vi "Change_Parameter.vi"(0 "Spinal Column In":T1={"Red MOT 88 Inputs"={"Active Device"="", "Active Channels"=[], "Waveform Parameters"=[], "Active Phases"=[], "Phase Times"=[], "Trigger Channel"=""}, "6704 Static Voltage Settings"={"Device Name"="", "Values"=[], "Nickname"=[], "Conversion"=[]}, "Instructions"=[], "Red MOT 87 Inputs"={"Active Device"="", "Active Channels"=[], "Waveform Parameters"=[], "Active Phases"=[], "Phase Times"=[], "Trigger Channel"=""}, "ODT Params"={"Waveform Parameters"=[], "Active Phases"=[], "Active Channels"=[], "Phase Times (s)"=[], "Active Device"="", "Trigger Channel"="", "Evaporation Phase"=0.0, "Evaporation Channel"=0.0}, "SR400 Settings"={"Channel A"={"Input"=0, "A Discriminator Level (V)"=0.0, "A Discriminator Slope"=enum."Rising", "A Gate Mode"=enum."CW", "A Gate Delay (s)"=0.0, "A Gate Width (s)"=0.0, "Scan Increment (s)"=0.0}, "Channel B"={"Input"=0, "B Discriminator Level (V)"=0.0, "B Discriminator Slope"=enum."Rising", "B Gate Mode"=enum."CW", "B Gate Delay (s)"=0.0, "B Gate Width (s)"=0.0, "Scan Increment (s)"=0.0}, "Channel T"={"Input"=0, "Trigger Level (V)"=0.0, "Trigger Slope"=enum."Rising", "T Discriminator Slope"=enum."Rising", "T Discriminator Level (V)"=0.0, "Trigger Preset"=0.0}, "N Periods"=0.0, "At N"=enum."Stop", "Counting Mode"=enum."A,B for T Preset", "GPIB Address"="", "Dwell Time (s)"=0.0, "Port 1 Mode"=0, "Port 1 Voltage"=0.0, "Port 1 Scan Increment"=0.0, "Port 2 Voltage"=0.0, "Port 2 Scan Increment"=0.0, "Port 2 Mode"=0, "Counter Toggle"=FALSE, "Pusleblater Settings"={"Loop Start Channel"=0.0, "Loop End Channel"=0.0, "Loop On"=FALSE}}, "Synth Controls"={"Channel Settings"=[], "Active Channels"=[], "COM Port"=""}, "Acquisition Parameters"={"Acquisition Mode"=enum."Reserved (0)", "Trigger Mode"=enum."Internal", "Frame \nTransfer"=FALSE, "Exposure Time (s)"=0.0, "Accumulation Cycle Time (s)"=0.0, "# Accumulations"=0, "# Kinetics"=0, "Kinetic Cycle Time (s)"=0.0, "Horizontal Bin Size"=0, "Vertical Bin Size"=0}, "Scan Parameters"={"Initial Values"=[], "Final Values"=[], "Step Sizes"=[], "Parameters to Change"=[], "Channels to Change"=[], "Number of Parameters to Scan"=0, "Parameter Nickname (no spaces)"=[], "Scan Base Name"="", "Raw_Data Folder"=path "", "ROI Parameters"={"Background Radius"=0.0, "Atom Radius"=0.0, "X Center"=0.0, "Y Center"=0.0}, "Drop Time (ms)"=0.0, "ODT VCA 1 Channel"=0.0, "ODT VCA 2 Channel"=0.0, "Phases To Change"=[], "Scan Pulseblaster Channel With Parameter"={"Change PB Time Toggle"=FALSE, "PB Channel"=0.0, "Parameter Number"=0.0}, "Preserve Waveform\nContinuity"=FALSE, "Generated Array Type"=enum."Custom Array From File", "Principle Quantum #"=0, "Angular Momentum"=enum."s", "Ramp Delay Channel"=0, "ODT Hold Channel"=0, "MCS ROI Min"=0, "MCS ROI Max"=0, "Master Batch Fourth Column"=0.0}, "MCS Parameters"={"Scan Length (Bins)"=0.0, "Dwell Time (s)"=0.0, "Gate Channel Settings"={"Threshold (V)"=0.0, "Edge"=enum."Falling", "Input Impedence"=enum."1k Ohm"}, "Trig Channel Settings"={"Threshold (V)"=0.0, "Edge"=enum."Falling", "Input Impedence"=enum."1k Ohm"}, "Input 1 Settings"={"Threshold (V)"=0.0, "Edge"=enum."Falling", "Input Impedence"=enum."1k Ohm"}, "Input 2 Settings"={"Threshold (V)"=0.0, "Edge"=enum."Falling", "Input Impedence"=enum."1k Ohm"}, "Number of Sweeps"=0, "Number of Sequential Cycles"=0.0, "Number of Sequences"=0.0, "Sweep Preset"=FALSE, "Sequential Mode"=FALSE, "DAC 1 Ramp Settings"={"Ramp Mode"=enum."Fixed", "Ramp Start Value (V)"=0.0, "Ramp Length (Steps)"=0, "Step Width (bins)"=0, "Step Size (V)"=0.0}, "DAC 2 Output (V)"=0.0, "SYNC Output"=enum."40 MHz Clock", "ROI Min"=0, "ROI Max"=0, "Dual MCS Mode"=FALSE, "DAC 2 Toggle"=FALSE, "MCS on/off"=FALSE, "ROI Max 2"=1, "ROI Min 2"=0}, "PicoScope"={"Channel A Settings"={"Enabled"=FALSE, "Coupling"=0, "Range"=0, "Analogue Offset"=0.0}, "Channel B Settings"={"Enabled"=FALSE, "Coupling"=0, "Range"=0, "Analogue Offset"=0.0}, "Trigger Options"={"Trigger Enabled"=FALSE, "Trigger Source"=enum."Channel A", "Trigger Threshold (-5 to 5 V)"=0.0, "Trigger Slope"=0, "Trigger Delay (ms)"=0.0, "Auto Trigger Time (ms)"=0}, "Pico Scope Inititalization Settings"={"USB Power"=FALSE, "Use Serial Number"=FALSE, "Resolution"=0, "Serial Number"="", "Handle"=0}, "Use PicoScope?"=FALSE, "Acquisition Settings"={"Pre Trigger Time (s)"=0.0, "Post Trigger Time (s)"=0.0, "Resolution (s)"=0.0, "Four Channel Device"=FALSE, "Number of Captures"=0.0}}, "Random Interleave Controls"={"Subroutine A"=[], "Subroutine B"=[], "Interleave On"=FALSE, "Number of loops"=0, "Insert after instruction"=0, "Random"=FALSE}} {"Red MOT 88 Inputs"."Phase Times" format="%.0p"; "Red MOT 87 Inputs"."Phase Times" format="%.0p"; "ODT Params"."Evaporation Channel" min=0.0 max=1.0 step=1.0; "ODT Params"."Evaporation Phase" min=0.0 max=4.0 step=1.0; "ODT Params"."Phase Times (s)" format="%#_6p"; "SR400 Settings"."Port 2 Mode" items=["Scan"=1, "Fixed"=0]; "SR400 Settings"."Port 2 Scan Increment" min=-0.5 max=0.5; "SR400 Settings"."Port 2 Voltage" min=-10.0 max=10.0; "SR400 Settings"."Port 1 Scan Increment" min=-0.5 max=-0.5; "SR400 Settings"."Port 1 Voltage" min=-10.0 max=10.0; "SR400 Settings"."Port 1 Mode" items=["Scan"=1, "Fixed"=0]; "SR400 Settings"."Dwell Time (s)" min=0.002 max=60.0 format="%#_6p"; "SR400 Settings"."N Periods" min=1.0 max=2000.0 step=1.0; "SR400 Settings"."Channel T"."Trigger Preset" min=1.0 max=900000000000.0 format="%#_1e"; "SR400 Settings"."Channel T"."T Discriminator Level (V)" min=-0.3 max=0.3 format="%#_6p"; "SR400 Settings"."Channel T"."Trigger Level (V)" min=-2.0 max=2.0 format="%#_6p"; "SR400 Settings"."Channel T"."Input" items=["10 MHz", "Input 2", "Trig"]; "SR400 Settings"."Channel B"."Scan Increment (s)" min=0.0 max=0.09992 format="%#_6p"; "SR400 Settings"."Channel B"."B Gate Width (s)" min=5e-09 max=0.9992 format="%#_6p"; "SR400 Settings"."Channel B"."B Gate Delay (s)" min=0.0 max=0.9992 format="%#_6p"; "SR400 Settings"."Channel B"."B Discriminator Level (V)" min=-0.3 max=0.3 format="%#_6p"; "SR400 Settings"."Channel B"."Input" items=["Input 2"=2, "Input 1"=1]; "SR400 Settings"."Channel A"."Scan Increment (s)" min=0.0 max=0.09992 format="%#_6p"; "SR400 Settings"."Channel A"."A Gate Width (s)" min=5e-09 max=0.9992 format="%#_6p"; "SR400 Settings"."Channel A"."A Gate Delay (s)" min=0.0 max=0.9992 format="%#_6p"; "SR400 Settings"."Channel A"."A Discriminator Level (V)" min=-0.3 max=0.3 format="%#_6p"; "SR400 Settings"."Channel A"."Input" items=["Input 1", "10 MHz"]; "Acquisition Parameters"."Vertical Bin Size" items=["6"=6, "3"=3, "2"=2, "1"=1]; "Acquisition Parameters"."Horizontal Bin Size" items=["4"=4, "2"=2, "1"=1]; "Acquisition Parameters"."Kinetic Cycle Time (s)" format="%.2f"; "Acquisition Parameters"."# Kinetics" min=1; "Acquisition Parameters"."# Accumulations" min=1; "Acquisition Parameters"."Accumulation Cycle Time (s)" format="%.2f"; "Acquisition Parameters"."Exposure Time (s)" format="%.2f"; "Scan Parameters"."Drop Time (ms)" min=1.0; "Scan Parameters"."Number of Parameters to Scan" min=1; "MCS Parameters"."ROI Max 2" min=1; "MCS Parameters"."ROI Min 2" min=0; "MCS Parameters"."ROI Max" min=1; "MCS Parameters"."ROI Min" min=0; "MCS Parameters"."DAC 2 Output (V)" min=-10.0 max=10.0 step=0.00488; "MCS Parameters"."DAC 1 Ramp Settings"."Step Size (V)" min=0.0 max=10.0 step=0.00244 format="%#_4g"; "MCS Parameters"."DAC 1 Ramp Settings"."Step Width (bins)" min=1; "MCS Parameters"."DAC 1 Ramp Settings"."Ramp Length (Steps)" min=1; "MCS Parameters"."DAC 1 Ramp Settings"."Ramp Start Value (V)" min=0.0 max=10.0 step=0.00244; "MCS Parameters"."Number of Sweeps" min=0 format="%.0p"; "MCS Parameters"."Input 2 Settings"."Threshold (V)" min=-2.5 max=2.5 step=0.001; "MCS Parameters"."Input 1 Settings"."Threshold (V)" min=-2.5 max=2.5 step=0.001; "MCS Parameters"."Trig Channel Settings"."Threshold (V)" min=-2.5 max=2.5 step=0.001; "MCS Parameters"."Gate Channel Settings"."Threshold (V)" min=-2.5 max=2.5 step=0.001; "MCS Parameters"."Dwell Time (s)" min=1e-07 step=2.5e-08 format="%#_6p"; "MCS Parameters"."Scan Length (Bins)" min=64.0 max=524288.0 format="%#_7f"; "PicoScope"."Acquisition Settings"."Resolution (s)" min=8e-09 max=34.36 step=8e-09 format="%#_6p"; "PicoScope"."Acquisition Settings"."Post Trigger Time (s)" min=0.0 format="%#_6p"; "PicoScope"."Acquisition Settings"."Pre Trigger Time (s)" min=0.0 format="%#_6p"; "PicoScope"."Pico Scope Inititalization Settings"."Resolution" items=["8-bit", "12-bit", "14-bit", "15-bit (max. 2 ch.)", "16-bit (max. 1 ch.)"]; "PicoScope"."Trigger Options"."Trigger Slope" items=["Rising"=2, "Falling"=3]; "PicoScope"."Channel B Settings"."Range" items=["10 mV", "20 mV", "50 mV", "100 mV", "200 mV", "500 mV", "1 V", "2 V", "5 V", "10 V", "20 V", "50 V ", "100 V"]; "PicoScope"."Channel B Settings"."Coupling" items=["AC", "DC"]; "PicoScope"."Channel A Settings"."Range" items=["10 mV", "20 mV", "50 mV", "100 mV", "200 mV", "500 mV", "1 V", "2 V", "5 V", "10 V", "20 V", "50 V ", "100 V"]; "PicoScope"."Channel A Settings"."Coupling" items=["AC", "DC"]; "Random Interleave Controls"."Insert after instruction" min=0; "Random Interleave Controls"."Subroutine B"."Time (s)" min=5e-08 format="%.3p"; "Random Interleave Controls"."Subroutine B"."Op Code" items=["Continue", "Stop", "Loop", "End Loop", "JSR", "RTS", "Branch", "Long Delay", "Wait"]; "Random Interleave Controls"."Subroutine B"."Instruct Data" format="%.0p"; "Random Interleave Controls"."Subroutine A"."Time (s)" min=5e-08 format="%.3p"; "Random Interleave Controls"."Subroutine A"."Op Code" items=["Continue", "Stop", "Loop", "End Loop", "JSR", "RTS", "Branch", "Long Delay", "Wait"]; "Random Interleave Controls"."Subroutine A"."Instruct Data" format="%.0p"}, 5 "What To Change":T25=enum."Synth Frequency", 7 "Channel To Change":dbl, 9 "Phase To Change":dbl, 11 "Value":dbl, 12 "Scan Pulseblaster Channel With Parameter":T27, 13 "Current Parameter":i32, 14 "Waveform Continuity":bool) -> (6 "Spinal Column Out":T1={"Red MOT 88 Inputs"={"Active Device"="", "Active Channels"=[], "Waveform Parameters"=[], "Active Phases"=[], "Phase Times"=[], "Trigger Channel"=""}, "6704 Static Voltage Settings"={"Device Name"="", "Values"=[], "Nickname"=[], "Conversion"=[]}, "Instructions"=[], "Red MOT 87 Inputs"={"Active Device"="", "Active Channels"=[], "Waveform Parameters"=[], "Active Phases"=[], "Phase Times"=[], "Trigger Channel"=""}, "ODT Params"={"Waveform Parameters"=[], "Active Phases"=[], "Active Channels"=[], "Phase Times (s)"=[], "Active Device"="", "Trigger Channel"="", "Evaporation Phase"=0.0, "Evaporation Channel"=0.0}, "SR400 Settings"={"Channel A"={"Input"=0, "A Discriminator Level (V)"=0.0, "A Discriminator Slope"=enum."Rising", "A Gate Mode"=enum."CW", "A Gate Delay (s)"=0.0, "A Gate Width (s)"=0.0, "Scan Increment (s)"=0.0}, "Channel B"={"Input"=0, "B Discriminator Level (V)"=0.0, "B Discriminator Slope"=enum."Rising", "B Gate Mode"=enum."CW", "B Gate Delay (s)"=0.0, "B Gate Width (s)"=0.0, "Scan Increment (s)"=0.0}, "Channel T"={"Input"=0, "Trigger Level (V)"=0.0, "Trigger Slope"=enum."Rising", "T Discriminator Slope"=enum."Rising", "T Discriminator Level (V)"=0.0, "Trigger Preset"=0.0}, "N Periods"=0.0, "At N"=enum."Stop", "Counting Mode"=enum."A,B for T Preset", "GPIB Address"="", "Dwell Time (s)"=0.0, "Port 1 Mode"=0, "Port 1 Voltage"=0.0, "Port 1 Scan Increment"=0.0, "Port 2 Voltage"=0.0, "Port 2 Scan Increment"=0.0, "Port 2 Mode"=0, "Counter Toggle"=FALSE, "Pusleblater Settings"={"Loop Start Channel"=0.0, "Loop End Channel"=0.0, "Loop On"=FALSE}}, "Synth Controls"={"Channel Settings"=[], "Active Channels"=[], "COM Port"=""}, "Acquisition Parameters"={"Acquisition Mode"=enum."Reserved (0)", "Trigger Mode"=enum."Internal", "Frame \nTransfer"=FALSE, "Exposure Time (s)"=0.0, "Accumulation Cycle Time (s)"=0.0, "# Accumulations"=0, "# Kinetics"=0, "Kinetic Cycle Time (s)"=0.0, "Horizontal Bin Size"=0, "Vertical Bin Size"=0}, "Scan Parameters"={"Initial Values"=[], "Final Values"=[], "Step Sizes"=[], "Parameters to Change"=[], "Channels to Change"=[], "Number of Parameters to Scan"=0, "Parameter Nickname (no spaces)"=[], "Scan Base Name"="", "Raw_Data Folder"=path "", "ROI Parameters"={"Background Radius"=0.0, "Atom Radius"=0.0, "X Center"=0.0, "Y Center"=0.0}, "Drop Time (ms)"=0.0, "ODT VCA 1 Channel"=0.0, "ODT VCA 2 Channel"=0.0, "Phases To Change"=[], "Scan Pulseblaster Channel With Parameter"={"Change PB Time Toggle"=FALSE, "PB Channel"=0.0, "Parameter Number"=0.0}, "Preserve Waveform\nContinuity"=FALSE, "Generated Array Type"=enum."Custom Array From File", "Principle Quantum #"=0, "Angular Momentum"=enum."s", "Ramp Delay Channel"=0, "ODT Hold Channel"=0, "MCS ROI Min"=0, "MCS ROI Max"=0, "Master Batch Fourth Column"=0.0}, "MCS Parameters"={"Scan Length (Bins)"=0.0, "Dwell Time (s)"=0.0, "Gate Channel Settings"={"Threshold (V)"=0.0, "Edge"=enum."Falling", "Input Impedence"=enum."1k Ohm"}, "Trig Channel Settings"={"Threshold (V)"=0.0, "Edge"=enum."Falling", "Input Impedence"=enum."1k Ohm"}, "Input 1 Settings"={"Threshold (V)"=0.0, "Edge"=enum."Falling", "Input Impedence"=enum."1k Ohm"}, "Input 2 Settings"={"Threshold (V)"=0.0, "Edge"=enum."Falling", "Input Impedence"=enum."1k Ohm"}, "Number of Sweeps"=0, "Number of Sequential Cycles"=0.0, "Number of Sequences"=0.0, "Sweep Preset"=FALSE, "Sequential Mode"=FALSE, "DAC 1 Ramp Settings"={"Ramp Mode"=enum."Fixed", "Ramp Start Value (V)"=0.0, "Ramp Length (Steps)"=0, "Step Width (bins)"=0, "Step Size (V)"=0.0}, "DAC 2 Output (V)"=0.0, "SYNC Output"=enum."40 MHz Clock", "ROI Min"=0, "ROI Max"=0, "Dual MCS Mode"=FALSE, "DAC 2 Toggle"=FALSE, "MCS on/off"=FALSE, "ROI Max 2"=1, "ROI Min 2"=0}, "PicoScope"={"Channel A Settings"={"Enabled"=FALSE, "Coupling"=0, "Range"=0, "Analogue Offset"=0.0}, "Channel B Settings"={"Enabled"=FALSE, "Coupling"=0, "Range"=0, "Analogue Offset"=0.0}, "Trigger Options"={"Trigger Enabled"=FALSE, "Trigger Source"=enum."Channel A", "Trigger Threshold (-5 to 5 V)"=0.0, "Trigger Slope"=0, "Trigger Delay (ms)"=0.0, "Auto Trigger Time (ms)"=0}, "Pico Scope Inititalization Settings"={"USB Power"=FALSE, "Use Serial Number"=FALSE, "Resolution"=0, "Serial Number"="", "Handle"=0}, "Use PicoScope?"=FALSE, "Acquisition Settings"={"Pre Trigger Time (s)"=0.0, "Post Trigger Time (s)"=0.0, "Resolution (s)"=0.0, "Four Channel Device"=FALSE, "Number of Captures"=0.0}}, "Random Interleave Controls"={"Subroutine A"=[], "Subroutine B"=[], "Interleave On"=FALSE, "Number of loops"=0, "Insert after instruction"=0, "Random"=FALSE}} {"Red MOT 88 Inputs"."Phase Times" format="%.0p"; "Red MOT 87 Inputs"."Phase Times" format="%.0p"; "ODT Params"."Evaporation Channel" min=0.0 max=1.0 step=1.0; "ODT Params"."Evaporation Phase" min=0.0 max=4.0 step=1.0; "ODT Params"."Phase Times (s)" format="%#_6p"; "SR400 Settings"."Port 2 Mode" items=["Scan"=1, "Fixed"=0]; "SR400 Settings"."Port 2 Scan Increment" min=-0.5 max=0.5; "SR400 Settings"."Port 2 Voltage" min=-10.0 max=10.0; "SR400 Settings"."Port 1 Scan Increment" min=-0.5 max=-0.5; "SR400 Settings"."Port 1 Voltage" min=-10.0 max=10.0; "SR400 Settings"."Port 1 Mode" items=["Scan"=1, "Fixed"=0]; "SR400 Settings"."Dwell Time (s)" min=0.002 max=60.0 format="%#_6p"; "SR400 Settings"."N Periods" min=1.0 max=2000.0 step=1.0; "SR400 Settings"."Channel T"."Trigger Preset" min=1.0 max=900000000000.0 format="%#_1e"; "SR400 Settings"."Channel T"."T Discriminator Level (V)" min=-0.3 max=0.3 format="%#_6p"; "SR400 Settings"."Channel T"."Trigger Level (V)" min=-2.0 max=2.0 format="%#_6p"; "SR400 Settings"."Channel T"."Input" items=["10 MHz", "Input 2", "Trig"]; "SR400 Settings"."Channel B"."Scan Increment (s)" min=0.0 max=0.09992 format="%#_6p"; "SR400 Settings"."Channel B"."B Gate Width (s)" min=5e-09 max=0.9992 format="%#_6p"; "SR400 Settings"."Channel B"."B Gate Delay (s)" min=0.0 max=0.9992 format="%#_6p"; "SR400 Settings"."Channel B"."B Discriminator Level (V)" min=-0.3 max=0.3 format="%#_6p"; "SR400 Settings"."Channel B"."Input" items=["Input 2"=2, "Input 1"=1]; "SR400 Settings"."Channel A"."Scan Increment (s)" min=0.0 max=0.09992 format="%#_6p"; "SR400 Settings"."Channel A"."A Gate Width (s)" min=5e-09 max=0.9992 format="%#_6p"; "SR400 Settings"."Channel A"."A Gate Delay (s)" min=0.0 max=0.9992 format="%#_6p"; "SR400 Settings"."Channel A"."A Discriminator Level (V)" min=-0.3 max=0.3 format="%#_6p"; "SR400 Settings"."Channel A"."Input" items=["Input 1", "10 MHz"]; "Acquisition Parameters"."Vertical Bin Size" items=["6"=6, "3"=3, "2"=2, "1"=1]; "Acquisition Parameters"."Horizontal Bin Size" items=["4"=4, "2"=2, "1"=1]; "Acquisition Parameters"."Kinetic Cycle Time (s)" format="%.2f"; "Acquisition Parameters"."# Kinetics" min=1; "Acquisition Parameters"."# Accumulations" min=1; "Acquisition Parameters"."Accumulation Cycle Time (s)" format="%.2f"; "Acquisition Parameters"."Exposure Time (s)" format="%.2f"; "Scan Parameters"."Drop Time (ms)" min=1.0; "Scan Parameters"."Number of Parameters to Scan" min=1; "MCS Parameters"."ROI Max 2" min=1; "MCS Parameters"."ROI Min 2" min=0; "MCS Parameters"."ROI Max" min=1; "MCS Parameters"."ROI Min" min=0; "MCS Parameters"."DAC 2 Output (V)" min=-10.0 max=10.0 step=0.00488; "MCS Parameters"."DAC 1 Ramp Settings"."Step Size (V)" min=0.0 max=10.0 step=0.00244 format="%#_4g"; "MCS Parameters"."DAC 1 Ramp Settings"."Step Width (bins)" min=1; "MCS Parameters"."DAC 1 Ramp Settings"."Ramp Length (Steps)" min=1; "MCS Parameters"."DAC 1 Ramp Settings"."Ramp Start Value (V)" min=0.0 max=10.0 step=0.00244; "MCS Parameters"."Number of Sweeps" min=0 format="%.0p"; "MCS Parameters"."Input 2 Settings"."Threshold (V)" min=-2.5 max=2.5 step=0.001; "MCS Parameters"."Input 1 Settings"."Threshold (V)" min=-2.5 max=2.5 step=0.001; "MCS Parameters"."Trig Channel Settings"."Threshold (V)" min=-2.5 max=2.5 step=0.001; "MCS Parameters"."Gate Channel Settings"."Threshold (V)" min=-2.5 max=2.5 step=0.001; "MCS Parameters"."Dwell Time (s)" min=1e-07 step=2.5e-08 format="%#_6p"; "MCS Parameters"."Scan Length (Bins)" min=64.0 max=524288.0 format="%#_7f"; "PicoScope"."Acquisition Settings"."Resolution (s)" min=8e-09 max=34.36 step=8e-09 format="%#_6p"; "PicoScope"."Acquisition Settings"."Post Trigger Time (s)" min=0.0 format="%#_6p"; "PicoScope"."Acquisition Settings"."Pre Trigger Time (s)" min=0.0 format="%#_6p"; "PicoScope"."Pico Scope Inititalization Settings"."Resolution" items=["8-bit", "12-bit", "14-bit", "15-bit (max. 2 ch.)", "16-bit (max. 1 ch.)"]; "PicoScope"."Trigger Options"."Trigger Slope" items=["Rising"=2, "Falling"=3]; "PicoScope"."Channel B Settings"."Range" items=["10 mV", "20 mV", "50 mV", "100 mV", "200 mV", "500 mV", "1 V", "2 V", "5 V", "10 V", "20 V", "50 V ", "100 V"]; "PicoScope"."Channel B Settings"."Coupling" items=["AC", "DC"]; "PicoScope"."Channel A Settings"."Range" items=["10 mV", "20 mV", "50 mV", "100 mV", "200 mV", "500 mV", "1 V", "2 V", "5 V", "10 V", "20 V", "50 V ", "100 V"]; "PicoScope"."Channel A Settings"."Coupling" items=["AC", "DC"]; "Random Interleave Controls"."Insert after instruction" min=0; "Random Interleave Controls"."Subroutine B"."Time (s)" min=5e-08 format="%.3p"; "Random Interleave Controls"."Subroutine B"."Op Code" items=["Continue", "Stop", "Loop", "End Loop", "JSR", "RTS", "Branch", "Long Delay", "Wait"]; "Random Interleave Controls"."Subroutine B"."Instruct Data" format="%.0p"; "Random Interleave Controls"."Subroutine A"."Time (s)" min=5e-08 format="%.3p"; "Random Interleave Controls"."Subroutine A"."Op Code" items=["Continue", "Stop", "Loop", "End Loop", "JSR", "RTS", "Branch", "Long Delay", "Wait"]; "Random Interleave Controls"."Subroutine A"."Instruct Data" format="%.0p"}, 10 "Value Out":dbl)   [LabVIEW 2013]
uses:
  Controls/ScanParameters/ScanPBandParam.ctl
  Controls/ScanParameters/ParameterToChange.ctl
  2015.06.22_Rydberg_ExpControl/Controls/Spinal Column/spinal_column.ctl
  6733_Red_MOT/6733_control_panel.ctl
  6733_Red_MOT/6733_waveform_parameter_array.ctl
  6733_Red_MOT/6733_waveform_item.ctl
  6733_Red_MOT/6733_voltage_conversions.ctl
  Controls/6704/6704_static_voltages_control.ctl
  Controls/6704/static_voltage_conversions.ctl
  testing ground/6221 arb waveforms/6221_panel.ctl
  testing ground/6221 arb waveforms/6221_waveform_param.ctl
  Controls/SR400/SR400.ctl
  Controls/SR400/Channel A/channelA.ctl
  Controls/SR400/Channel A/channelA_inputs.ctl
  Controls/SR400/discrim_slope.ctl
  Controls/SR400/gate_mode.ctl
  Controls/SR400/Channel B/channelB.ctl
  Controls/SR400/Channel B/inputsB.ctl
  Controls/SR400/Channel T/channelT.ctl
  Controls/SR400/Channel T/inputsT.ctl
  Controls/Synth_409b/Synth_controls.ctl
  Controls/Synth_409b/synth_channel.ctl
  testing ground/AndorCamera/camera_controls.ctl
  testing ground/CameraTest/System Files/user.lib/atmcd32d.llb/AcquisitionMode_mode typedef.ctl
  testing ground/CameraTest/System Files/user.lib/atmcd32d.llb/TriggerMode_mode typedef.ctl
  Controls/ScanParameters/ScanParametersPanel.ctl
  Controls/ScanParameters/ROI_set.ctl
  Controls/MCS/mcs_control_panel.ctl
  Controls/MCS/mcs_channel.ctl
  Controls/MCS/ramp_control.ctl
  Controls/PicoScope/pico_control_panel.ctl
  Controls/PicoScope/pico_channel_settings.ctl
  Controls/PicoScope/pico_trigger.ctl
  Controls/PicoScope/pico_init_settings.ctl
  2015.06.22_Rydberg_ExpControl/Controls/PulseBlaster/interleaveControls.ctl
panel:
  # "(0) 689 Center Freq"
  # "(1) 689 Dither Amp"
  # "(2) 689 Power Lock"
  # "(3) Red MOT Field Grad"
  # "(0) 689 Center Freq"
  # "(1) 689 Dither Amp"
  # "(2) 689 Power Lock"
  # "(3) Red MOT Field Grad"
  # "Select a PB Channel to set with a phase time\nfor evaporation or whatever"
  # "1"
  # "2"
  # "3"
  # "4"
  # "5"
  # "6"
  # "7"
  # "8"
  # "9"
  # "10"
  # "11"
  # "12"
  # "13"
  # "14"
  # "15"
  # "16"
  # "17"
  # "18"
  # "19"
  # "20"
  # "21"
  # "22"
  # "23"
  # "24"
  # "1"
  # "2"
  # "3"
  # "4"
  # "5"
  # "6"
  # "7"
  # "8"
  # "9"
  # "10"
  # "11"
  # "12"
  # "13"
  # "14"
  # "15"
  # "16"
  # "17"
  # "18"
  # "19"
  # "20"
  # "21"
  # "22"
  # "23"
  # "24"
  # "(0) 689 Center Freq"
  # "(1) 689 Dither Amp"
  # "(2) 689 Power Lock"
  # "(3) Red MOT Field Grad"
  # "(0) 689 Center Freq"
  # "(1) 689 Dither Amp"
  # "(2) 689 Power Lock"
  # "(3) Red MOT Field Grad"
  # "Select a PB Channel to set with a phase time\nfor evaporation or whatever"
  # "1"
  # "2"
  # "3"
  # "4"
  # "5"
  # "6"
  # "7"
  # "8"
  # "9"
  # "10"
  # "11"
  # "12"
  # "13"
  # "14"
  # "15"
  # "16"
  # "17"
  # "18"
  # "19"
  # "20"
  # "21"
  # "22"
  # "23"
  # "24"
  # "1"
  # "2"
  # "3"
  # "4"
  # "5"
  # "6"
  # "7"
  # "8"
  # "9"
  # "10"
  # "11"
  # "12"
  # "13"
  # "14"
  # "15"
  # "16"
  # "17"
  # "18"
  # "19"
  # "20"
  # "21"
  # "22"
  # "23"
  # "24"
  # "Select a PB Channel to set with a phase time\nfor evaporation or whatever"
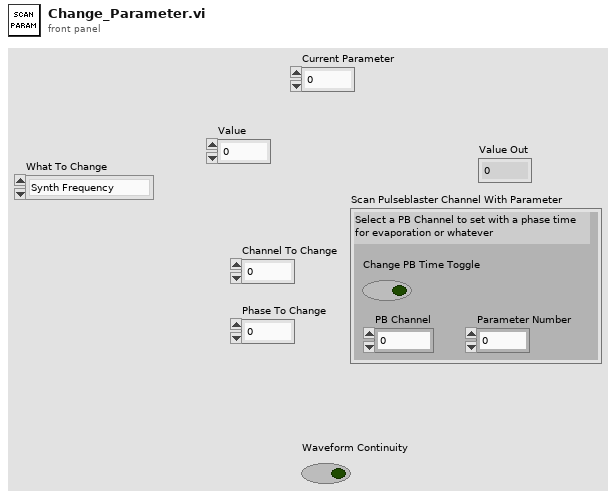
[diagram p1: front panel]
types:
  T1 = typedef "spinal_column.ctl" = cluster{"Red MOT 88 Inputs":T2, "6704 Static Voltage Settings":T6, "Instructions":cluster{"Instruct Data":i32, "Op Code":i32, "Flags":bool[], "Comments":string, "Time (s)":dbl}[], "Red MOT 87 Inputs":T2, "ODT Params":T8, "SR400 Settings":T10, "Synth Controls":T19, "Acquisition Parameters":T21, "Scan Parameters":T24, "MCS Parameters":T28, "PicoScope":T31, "Random Interleave Controls":T35}
  T2 = typedef "6733_control_panel.ctl" = cluster{"Active Device":string, "Active Channels":bool[], "Waveform Parameters":T3, "Active Phases":bool[], "Phase Times":dbl[], "Trigger Channel":tag}
  T3 = typedef "6733_waveform_parameter_array.ctl" = T4[][]
  T4 = typedef "6733_waveform_item.ctl" = cluster{"Functional Form":enum16{"Polynomial", "Exponential"}, "Start Voltage":dbl, "End Voltage":dbl, "Degree":i8, "Nickname":string, "Conversion":T5}
  T5 = typedef "6733_voltage_conversions.ctl" = enum16{"B Field Grad (G/cm)", "Red AOM Center Freq (MHz)", "Red Dither Pk(kHz)", "Red Power (mW)", "Volts"}
  T6 = typedef "6704_static_voltages_control.ctl" = cluster{"Device Name":string, "Values":dbl[], "Nickname":string[], "Conversion":T7[]}
  T7 = typedef "static_voltage_conversions.ctl" = enum16{"Volts", "ODT Power Lock (W)", "Sat Abs Detuning (MHz)", "Blue Mot Power Lock (mW)"}
  T8 = typedef "6221_panel.ctl" = cluster{"Waveform Parameters":T9[][], "Active Phases":bool[], "Active Channels":bool[], "Phase Times (s)":dbl[], "Active Device":string, "Trigger Channel":tag, "Evaporation Phase":dbl, "Evaporation Channel":dbl}
  T9 = typedef "6221_waveform_param.ctl" = cluster{"Initial Value":dbl, "Final Value":dbl, "Tau":dbl, "Eta":dbl, "Nickname":string, "Enum":enum16{"Volts to Volts", "Power Law", "Evaporation Formula"}}
  T10 = typedef "SR400.ctl" = cluster{"Channel A":T11, "Channel B":T15, "Channel T":T17, "N Periods":dbl, "At N":enum16{"Stop", "Start"}, "Counting Mode":enum16{"A,B for T Preset", "A-B for T Preset", "A+B for T Preset"}, "GPIB Address":string, "Dwell Time (s)":dbl, "Port 1 Mode":i32, "Port 1 Voltage":dbl, "Port 1 Scan Increment":dbl, "Port 2 Voltage":dbl, "Port 2 Scan Increment":dbl, "Port 2 Mode":i32, "Counter Toggle":bool, "Pusleblater Settings":cluster{"Loop Start Channel":dbl, "Loop End Channel":dbl, "Loop On":bool}}
  T11 = typedef "channelA.ctl" = cluster{"Input":T12, "A Discriminator Level (V)":dbl, "A Discriminator Slope":T13, "A Gate Mode":T14, "A Gate Delay (s)":dbl, "A Gate Width (s)":dbl, "Scan Increment (s)":dbl}
  T12 = typedef "channelA_inputs.ctl" = u16
  T13 = typedef "discrim_slope.ctl" = enum16{"Rising", "Falling"}
  T14 = typedef "gate_mode.ctl" = enum16{"CW", "Fixed", "Scan"}
  T15 = typedef "channelB.ctl" = cluster{"Input":T16, "B Discriminator Level (V)":dbl, "B Discriminator Slope":T13, "B Gate Mode":T14, "B Gate Delay (s)":dbl, "B Gate Width (s)":dbl, "Scan Increment (s)":dbl}
  T16 = typedef "inputsB.ctl" = u16
  T17 = typedef "channelT.ctl" = cluster{"Input":T18, "Trigger Level (V)":dbl, "Trigger Slope":T13, "T Discriminator Slope":T13, "T Discriminator Level (V)":dbl, "Trigger Preset":dbl}
  T18 = typedef "inputsT.ctl" = u16
  T19 = typedef "Synth_controls.ctl" = cluster{"Channel Settings":T20[], "Active Channels":bool[], "COM Port":refnum<visa-resource-name>}
  T20 = typedef "synth_channel.ctl" = cluster{"Voltage (Pk-Pk) ":dbl, "Frequency (MHz)":dbl, "Phase (deg)":dbl, "Nickname":string}
  T21 = typedef "camera_controls.ctl" = cluster{"Acquisition Mode":T22, "Trigger Mode":T23, "Frame \nTransfer":bool, "Exposure Time (s)":sgl, "Accumulation Cycle Time (s)":sgl, "# Accumulations":i32, "# Kinetics":i32, "Kinetic Cycle Time (s)":sgl, "Horizontal Bin Size":i32, "Vertical Bin Size":i32}
  T22 = typedef "AcquisitionMode_mode typedef.ctl" = enum16{"Reserved (0)", "Single Scan", "Accumulate", "Kinetics", "Fast Kinetics", "Run Till Abort", "Reserved (6)", "Reserved (7)", "Reserved (8)", "Time Delayed Integration"}
  T23 = typedef "TriggerMode_mode typedef.ctl" = enum16{"Internal", "External", "N/A (2)", "N/A (3)", "N/A (4)", "N/A (5)", "External Start", "External Exposure (Bulb)", "N/A (8)", "External FVB EM", "Software", "N/A (11)", "External Charge Shifting"}
  T24 = typedef "ScanParametersPanel.ctl" = cluster{"Initial Values":dbl[], "Final Values":dbl[], "Step Sizes":dbl[], "Parameters to Change":T25[], "Channels to Change":dbl[], "Number of Parameters to Scan":i32, "Parameter Nickname (no spaces)":string[], "Scan Base Name":string, "Raw_Data Folder":path, "ROI Parameters":T26, "Drop Time (ms)":dbl, "ODT VCA 1 Channel":dbl, "ODT VCA 2 Channel":dbl, "Phases To Change":dbl[], "Scan Pulseblaster Channel With Parameter":T27, "Preserve Waveform\nContinuity":bool, "Generated Array Type":enum16{"Custom Array From File", "Default (old way)"}, "Principle Quantum #":i32, "Angular Momentum":enum16{"s", "p", "d", "f", "g", "h"}, "Ramp Delay Channel":i32, "ODT Hold Channel":i32, "MCS ROI Min":i32, "MCS ROI Max":i32, "Master Batch Fourth Column":dbl}
  T25 = typedef "ParameterToChange.ctl" = enum16{"Subroutine A Time", "Subroutine B Time", "Synth Amplitude", "Synth Frequency", "Synth Phase", "ODT Params Phase Time", "ODT Params Tau", "ODT Params Final Voltage", "ODT Params Initial Voltage", "ODT Params Eta", "Red Mot 88 Phase Time", "Red Mot 87 Phase Time", "Red Mot 88 Final Voltage", "Red Mot 88 Initial Voltage", "Red Mot 87 Final Voltage", "Red Mot 87 Initial Voltage", "PulseBlaster", "Static Voltage"}
  T26 = typedef "ROI_set.ctl" = cluster{"Background Radius":dbl, "Atom Radius":dbl, "X Center":dbl, "Y Center":dbl}
  T27 = typedef "ScanPBandParam.ctl" = cluster{"Change PB Time Toggle":bool, "PB Channel":dbl, "Parameter Number":dbl}
  T28 = typedef "mcs_control_panel.ctl" = cluster{"Scan Length (Bins)":dbl, "Dwell Time (s)":dbl, "Gate Channel Settings":T29, "Trig Channel Settings":T29, "Input 1 Settings":T29, "Input 2 Settings":T29, "Number of Sweeps":i32, "Number of Sequential Cycles":dbl, "Number of Sequences":dbl, "Sweep Preset":bool, "Sequential Mode":bool, "DAC 1 Ramp Settings":T30, "DAC 2 Output (V)":dbl, "SYNC Output":enum16{"40 MHz Clock", "Gate Disc Signal", "Trigger Disc Signal", "Counter 1 Disc Signal", "Counter 2 Disc Signal", "Definitely Not Used", "Not Used", "1 kHz Signal", "Also Not Used", "MCS On/Off", "End of Time Bin", "Ramp Increment Trig", "Step Count Trigger", "'GO'-Line", "Ramp Down Trigger", "Logic 1"}, "ROI Min":i32, "ROI Max":i32, "Dual MCS Mode":bool, "DAC 2 Toggle":bool, "MCS on/off":bool, "ROI Max 2":i32, "ROI Min 2":i32}
  T29 = typedef "mcs_channel.ctl" = cluster{"Threshold (V)":dbl, "Edge":enum16{"Falling", "Rising"}, "Input Impedence":enum16{"1k Ohm", "50 Ohm"}}
  T30 = typedef "ramp_control.ctl" = cluster{"Ramp Mode":enum16{"Fixed", "Triangle", "Sawtooth"}, "Ramp Start Value (V)":dbl, "Ramp Length (Steps)":i32, "Step Width (bins)":i32, "Step Size (V)":dbl}
  T31 = typedef "pico_control_panel.ctl" = cluster{"Channel A Settings":T32, "Channel B Settings":T32, "Trigger Options":T33, "Pico Scope Inititalization Settings":T34, "Use PicoScope?":bool, "Acquisition Settings":cluster{"Pre Trigger Time (s)":dbl, "Post Trigger Time (s)":dbl, "Resolution (s)":dbl, "Four Channel Device":bool, "Number of Captures":dbl}}
  T32 = typedef "pico_channel_settings.ctl" = cluster{"Enabled":bool, "Coupling":i16, "Range":u16, "Analogue Offset":sgl}
  T33 = typedef "pico_trigger.ctl" = cluster{"Trigger Enabled":bool, "Trigger Source":enum16{"Channel A", "Channel B", "Channel C", "Channel D", "Ext."}, "Trigger Threshold (-5 to 5 V)":dbl, "Trigger Slope":u16, "Trigger Delay (ms)":dbl, "Auto Trigger Time (ms)":i16}
  T34 = typedef "pico_init_settings.ctl" = cluster{"USB Power":bool, "Use Serial Number":bool, "Resolution":i32, "Serial Number":string, "Handle":i16}
  T35 = typedef "interleaveControls.ctl" = cluster{"Subroutine A":cluster{"Instruct Data":i32, "Op Code":i32, "Flags":bool[], "Comments":string, "Time (s)":dbl}[], "Subroutine B":cluster{"Instruct Data":i32, "Op Code":i32, "Flags":bool[], "Comments":string, "Time (s)":dbl}[], "Interleave On":bool, "Number of loops":i32, "Insert after instruction":i32, "Random":bool}
  T36 = cluster{"Instruct Data":i32, "Op Code":i32, "Flags":bool[], "Comments":string, "Time (s)":dbl}[]
  T37 = cluster{"Instruct Data":i32, "Op Code":i32, "Flags":bool[], "Comments":string, "Time (s)":dbl}
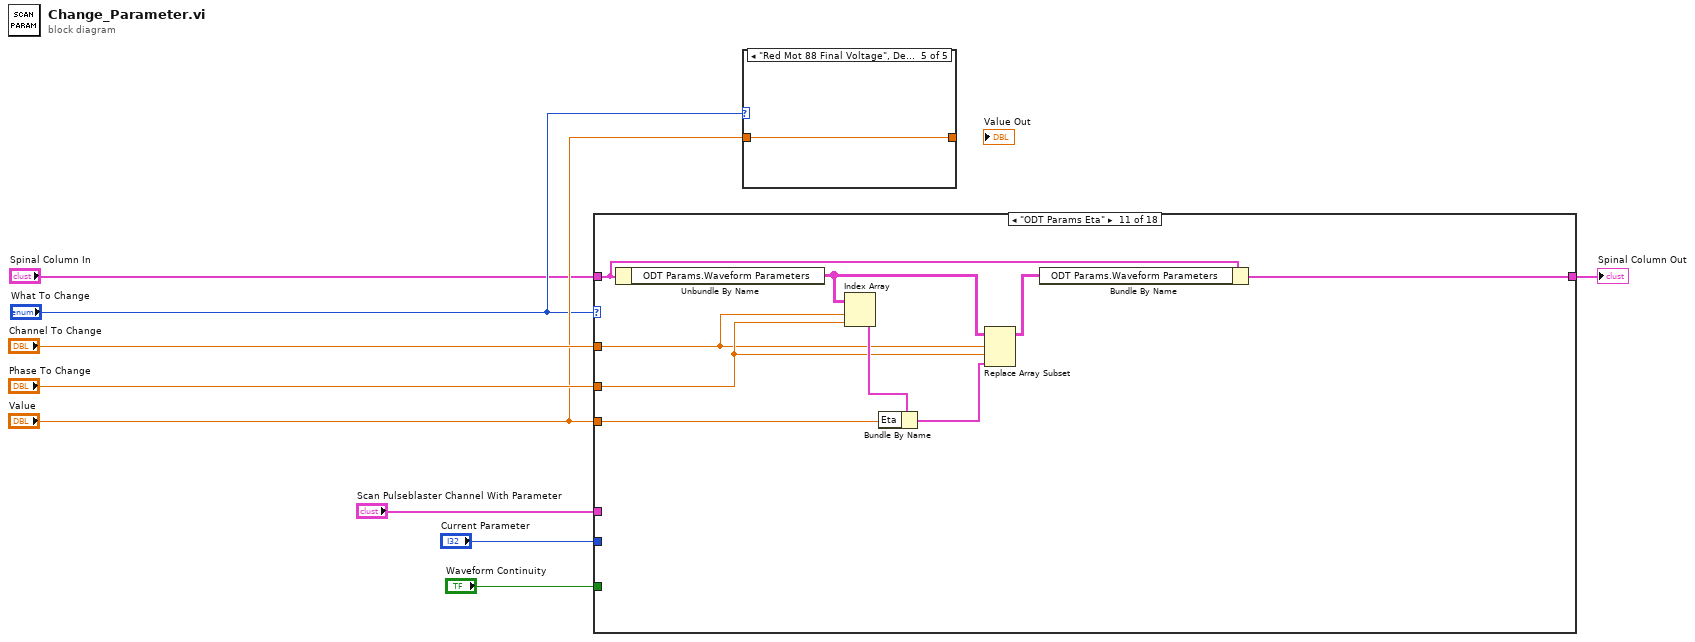
[diagram p0: block diagram]
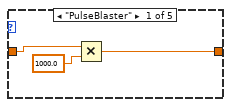
[diagram p2: hidden frame]
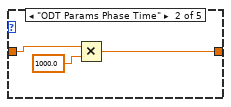
[diagram p3: hidden frame]
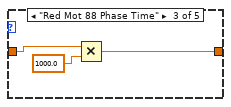
[diagram p4: hidden frame]
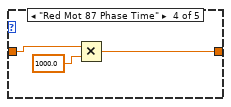
[diagram p5: hidden frame]
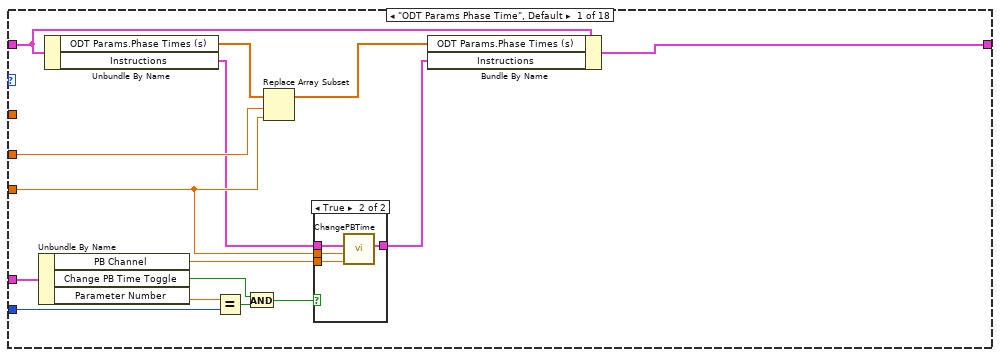
[diagram p6: hidden frame]
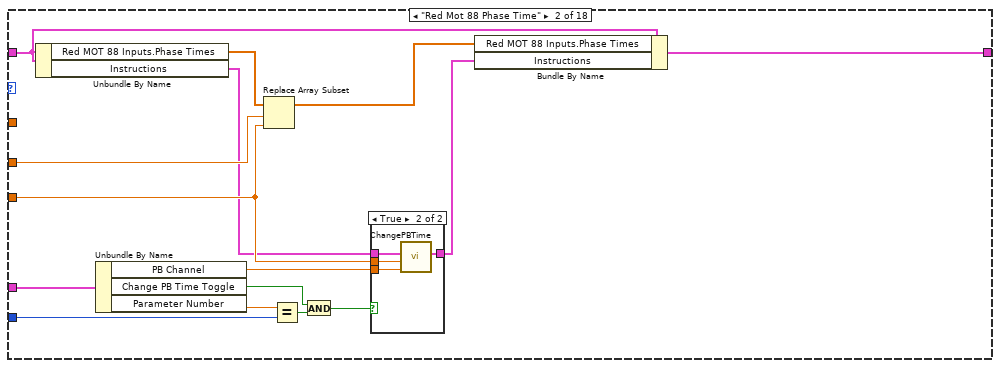
[diagram p8: hidden frame]
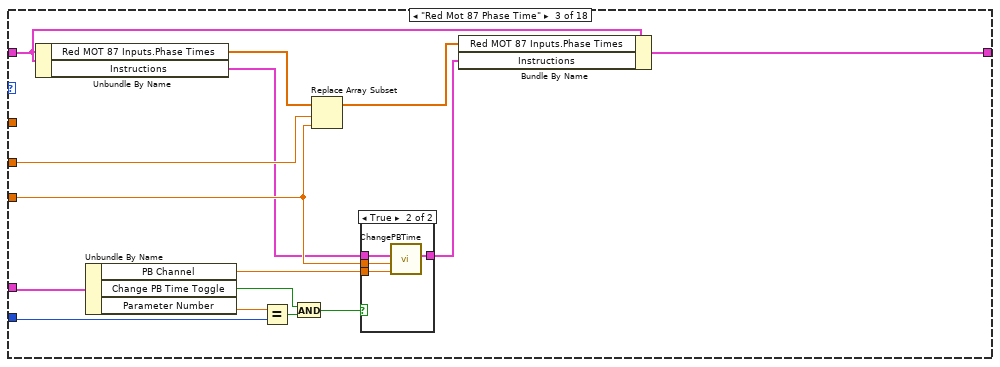
[diagram p10: hidden frame]
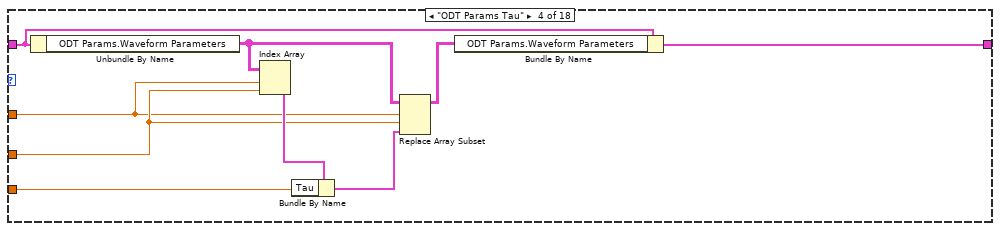
[diagram p12: hidden frame]
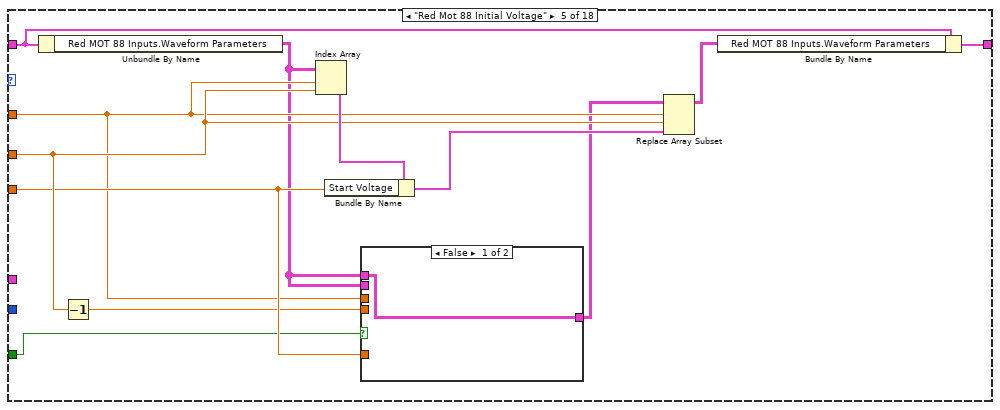
[diagram p13: hidden frame]
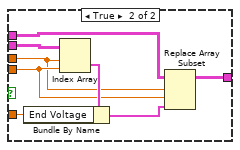
[diagram p14: hidden frame]
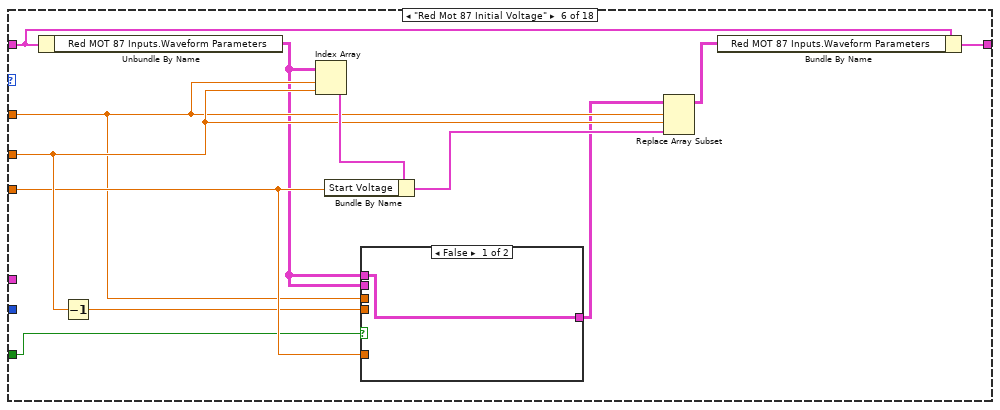
[diagram p15: hidden frame]
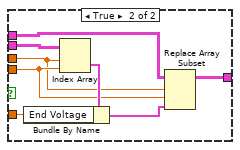
[diagram p16: hidden frame]
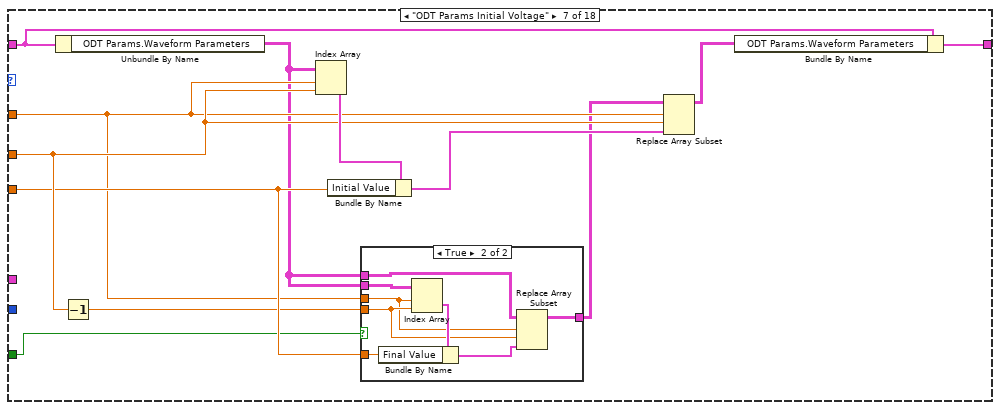
[diagram p17: hidden frame]
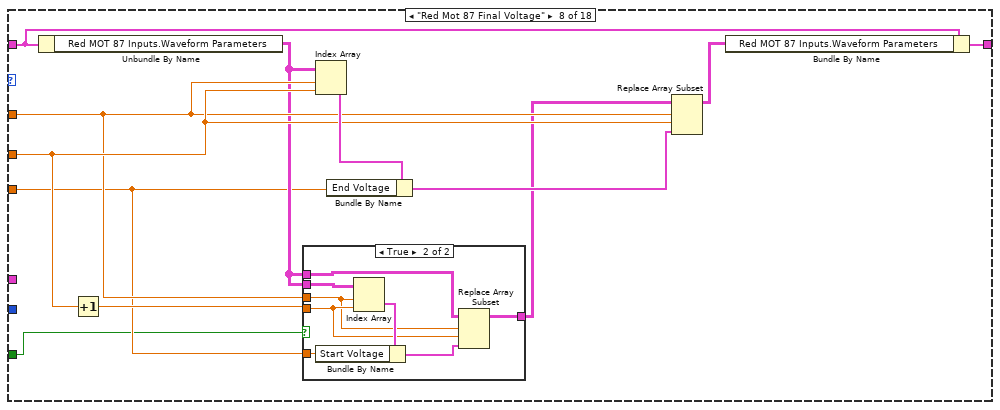
[diagram p19: hidden frame]
diagram:
  n1 = case shown="\"ODT Params Eta\"" "What To Change" {
    tunnel: "Spinal Column In" -> [w24 w44 w64 w78 w90 w111 w132 w153 w174 w195 w213 w221 w229 w237 w243 w246 w254 w262]
    tunnel: "Channel To Change" -> [_ _ _ w71 w83 w104 w125 w146 w167 w188 w206 w216 w224 w232 w240 w248 w256 w264]
    tunnel: "Phase To Change" -> [w21 w41 w61 w72 w85 w106 w127 w148 w169 w190 w207 _ _ _ _ _ _ _]
    tunnel: "Value" -> [w12 w32 w52 w75 w84 w105 w126 w144 w165 w186 w210 w219 w227 w235 w239 w250 w258 w266]
    tunnel: [w23 w43 w63 w77 w89 w110 w131 w152 w173 w194 w212 w220 w228 w236 w242 w244 w252 w260] -> w1
    tunnel: "Scan Pulseblaster Channel With Parameter" -> [w19 w35 w55 _ _ _ _ _ _ _ _ _ _ _ _ _ _ _]
    tunnel: "Current Parameter" -> [w15 w34 w54 _ _ _ _ _ _ _ _ _ _ _ _ _ _ _]
    tunnel: "Waveform Continuity" -> [_ _ _ _ w79 w100 w121 w143 w164 w185 _ _ _ _ _ _ _ _]
    frame "ODT Params Phase Time", Default {
      n2 = Unbundle By Name(w19) -> ("PB Channel"=w13:dbl, "Change PB Time Toggle"=w17:bool, "Parameter Number"=w16:dbl)
      n3 = Unbundle By Name(w24) -> ("ODT Params.Phase Times (s)"=w22:dbl[], "Instructions"=w10:T36)
      n4 = Equal?(x=w16, y=w15) -> (x = y?=w14:bool)
      n5 = And(x=w17, y=w14) -> (x .and. y?=w18:bool)
      n6 = Replace Array Subset(array=w22, new element=w12, index=w21) -> (w20:dbl[])
      n7 = case shown="True" w18 {
        tunnel: w13 -> [_ w29]
        tunnel: w12 -> [_ w28]
        tunnel: [w25 w27] -> w11
        tunnel: w10 -> [w25 w26]
        frame False {
        }
        frame True {
          n8 = call "ChangePBTime.vi"("Instruction to change"=w29, "Time (s)"=w28, "Instructions"=w26) -> ("Instructions out"=w27:T36)  [unwired: 7 in]
        }
      }
      n9 = Bundle By Name(cluster=w24, "ODT Params.Phase Times (s)"=w20, "Instructions"=w11) -> (w23:T1)
    }
    frame "Red Mot 88 Phase Time" {
      n10 = Unbundle By Name(w44) -> ("Red MOT 88 Inputs.Phase Times"=w42:dbl[], "Instructions"=w31:T36)
      n11 = Unbundle By Name(w35) -> ("PB Channel"=w36:dbl, "Change PB Time Toggle"=w39:bool, "Parameter Number"=w38:dbl)
      n12 = Replace Array Subset(array=w42, new element=w32, index=w41) -> (w40:dbl[])
      n13 = Equal?(x=w38, y=w34) -> (x = y?=w37:bool)
      n14 = And(x=w39, y=w37) -> (x .and. y?=w33:bool)
      n15 = case shown="True" w33 {
        tunnel: w36 -> [_ w49]
        tunnel: w32 -> [_ w48]
        tunnel: [w45 w47] -> w30
        tunnel: w31 -> [w45 w46]
        frame False {
        }
        frame True {
          n16 = call "ChangePBTime.vi"("Instruction to change"=w49, "Time (s)"=w48, "Instructions"=w46) -> ("Instructions out"=w47:T36)  [unwired: 7 in]
        }
      }
      n17 = Bundle By Name(cluster=w44, "Red MOT 88 Inputs.Phase Times"=w40, "Instructions"=w30) -> (w43:T1)
    }
    frame "Red Mot 87 Phase Time" {
      n18 = Unbundle By Name(w64) -> ("Red MOT 87 Inputs.Phase Times"=w62:dbl[], "Instructions"=w51:T36)
      n19 = Unbundle By Name(w55) -> ("PB Channel"=w56:dbl, "Change PB Time Toggle"=w59:bool, "Parameter Number"=w58:dbl)
      n20 = Equal?(x=w58, y=w54) -> (x = y?=w57:bool)
      n21 = And(x=w59, y=w57) -> (x .and. y?=w53:bool)
      n22 = Replace Array Subset(array=w62, new element=w52, index=w61) -> (w60:dbl[])
      n23 = case shown="True" w53 {
        tunnel: w56 -> [_ w69]
        tunnel: w52 -> [_ w68]
        tunnel: [w65 w67] -> w50
        tunnel: w51 -> [w65 w66]
        frame False {
        }
        frame True {
          n24 = call "ChangePBTime.vi"("Instruction to change"=w69, "Time (s)"=w68, "Instructions"=w66) -> ("Instructions out"=w67:T36)  [unwired: 7 in]
        }
      }
      n25 = Bundle By Name(cluster=w64, "Red MOT 87 Inputs.Phase Times"=w60, "Instructions"=w50) -> (w63:T1)
    }
    frame "ODT Params Tau" {
      n26 = Unbundle By Name(w78) -> ("ODT Params.Waveform Parameters"=w73:T9[][])
      n27 = Index Array(array=w73, index (row)=w71, index (col)=w72) -> (element=w76:T9)
      n28 = Bundle By Name(cluster=w76, "Tau"=w75) -> (w74:T9)
      n29 = Replace Array Subset(array=w73, new element=w74, index (row)=w71, index (col)=w72) -> (w70:T9[][])
      n30 = Bundle By Name(cluster=w78, "ODT Params.Waveform Parameters"=w70) -> (w77:T1)
    }
    frame "Red Mot 88 Initial Voltage" {
      n31 = Unbundle By Name(w90) -> ("Red MOT 88 Inputs.Waveform Parameters"=w81:T3)
      n32 = Decrement(x=w85) -> (x-1=w82:dbl)
      n33 = Index Array(array=w81, index (row)=w83, index (col)=w85) -> (element=w88:T4)
      n34 = Bundle By Name(cluster=w88, "Start Voltage"=w84) -> (w87:T4)
      n35 = case shown="False" w79 {
        tunnel: w81 -> [_ w98]
        tunnel: w84 -> [_ w97]
        tunnel: w83 -> [_ w93]
        tunnel: w82 -> [_ w94]
        tunnel: w81 -> [w91 w95]
        tunnel: [w91 w92] -> w80
        frame False {
        }
        frame True {
          n36 = Index Array(array=w98, index (row)=w93, index (col)=w94) -> (element=w99:T4)
          n37 = Bundle By Name(cluster=w99, "End Voltage"=w97) -> (w96:T4)
          n38 = Replace Array Subset(array=w95, new element=w96, index (row)=w93, index (col)=w94) -> (w92:T3)
        }
      }
      n39 = Replace Array Subset(array=w80, new element=w87, index (row)=w83, index (col)=w85) -> (w86:T3)
      n40 = Bundle By Name(cluster=w90, "Red MOT 88 Inputs.Waveform Parameters"=w86) -> (w89:T1)
    }
    frame "Red Mot 87 Initial Voltage" {
      n41 = Unbundle By Name(w111) -> ("Red MOT 87 Inputs.Waveform Parameters"=w102:T3)
      n42 = Decrement(x=w106) -> (x-1=w103:dbl)
      n43 = Index Array(array=w102, index (row)=w104, index (col)=w106) -> (element=w109:T4)
      n44 = Bundle By Name(cluster=w109, "Start Voltage"=w105) -> (w108:T4)
      n45 = case shown="False" w100 {
        tunnel: w102 -> [_ w119]
        tunnel: w105 -> [_ w118]
        tunnel: w104 -> [_ w114]
        tunnel: w103 -> [_ w115]
        tunnel: w102 -> [w112 w116]
        tunnel: [w112 w113] -> w101
        frame False {
        }
        frame True {
          n46 = Index Array(array=w119, index (row)=w114, index (col)=w115) -> (element=w120:T4)
          n47 = Bundle By Name(cluster=w120, "End Voltage"=w118) -> (w117:T4)
          n48 = Replace Array Subset(array=w116, new element=w117, index (row)=w114, index (col)=w115) -> (w113:T3)
        }
      }
      n49 = Replace Array Subset(array=w101, new element=w108, index (row)=w104, index (col)=w106) -> (w107:T3)
      n50 = Bundle By Name(cluster=w111, "Red MOT 87 Inputs.Waveform Parameters"=w107) -> (w110:T1)
    }
    frame "ODT Params Initial Voltage" {
      n51 = Unbundle By Name(w132) -> ("ODT Params.Waveform Parameters"=w123:T9[][])
      n52 = Decrement(x=w127) -> (x-1=w124:dbl)
      n53 = Index Array(array=w123, index (row)=w125, index (col)=w127) -> (element=w130:T9)
      n54 = Bundle By Name(cluster=w130, "Initial Value"=w126) -> (w129:T9)
      n55 = case shown="True" w121 {
        tunnel: w123 -> [_ w140]
        tunnel: w126 -> [_ w139]
        tunnel: w125 -> [_ w135]
        tunnel: w124 -> [_ w136]
        tunnel: w123 -> [w133 w137]
        tunnel: [w133 w134] -> w122
        frame False {
        }
        frame True {
          n56 = Index Array(array=w140, index (row)=w135, index (col)=w136) -> (element=w141:T9)
          n57 = Bundle By Name(cluster=w141, "Final Value"=w139) -> (w138:T9)
          n58 = Replace Array Subset(array=w137, new element=w138, index (row)=w135, index (col)=w136) -> (w134:T9[][])
        }
      }
      n59 = Replace Array Subset(array=w122, new element=w129, index (row)=w125, index (col)=w127) -> (w128:T9[][])
      n60 = Bundle By Name(cluster=w132, "ODT Params.Waveform Parameters"=w128) -> (w131:T1)
    }
    frame "Red Mot 87 Final Voltage" {
      n61 = Unbundle By Name(w153) -> ("Red MOT 87 Inputs.Waveform Parameters"=w145:T3)
      n62 = Increment(x=w148) -> (x+1=w147:dbl)
      n63 = case shown="True" w143 {
        tunnel: w145 -> [_ w161]
        tunnel: w144 -> [_ w160]
        tunnel: w146 -> [_ w156]
        tunnel: w147 -> [_ w157]
        tunnel: w145 -> [w154 w158]
        tunnel: [w154 w155] -> w142
        frame False {
        }
        frame True {
          n64 = Index Array(array=w161, index (row)=w156, index (col)=w157) -> (element=w162:T4)
          n65 = Bundle By Name(cluster=w162, "Start Voltage"=w160) -> (w159:T4)
          n66 = Replace Array Subset(array=w158, new element=w159, index (row)=w156, index (col)=w157) -> (w155:T3)
        }
      }
      n67 = Index Array(array=w145, index (row)=w146, index (col)=w148) -> (element=w151:T4)
      n68 = Bundle By Name(cluster=w151, "End Voltage"=w144) -> (w150:T4)
      n69 = Replace Array Subset(array=w142, new element=w150, index (row)=w146, index (col)=w148) -> (w149:T3)
      n70 = Bundle By Name(cluster=w153, "Red MOT 87 Inputs.Waveform Parameters"=w149) -> (w152:T1)
    }
    frame "Red Mot 88 Final Voltage" {
      n71 = Unbundle By Name(w174) -> ("Red MOT 88 Inputs.Waveform Parameters"=w166:T3)
      n72 = Increment(x=w169) -> (x+1=w168:dbl)
      n73 = case shown="True" w164 {
        tunnel: w166 -> [_ w182]
        tunnel: w165 -> [_ w181]
        tunnel: w167 -> [_ w177]
        tunnel: w168 -> [_ w178]
        tunnel: w166 -> [w175 w179]
        tunnel: [w175 w176] -> w163
        frame False {
        }
        frame True {
          n74 = Index Array(array=w182, index (row)=w177, index (col)=w178) -> (element=w183:T4)
          n75 = Bundle By Name(cluster=w183, "Start Voltage"=w181) -> (w180:T4)
          n76 = Replace Array Subset(array=w179, new element=w180, index (row)=w177, index (col)=w178) -> (w176:T3)
        }
      }
      n77 = Index Array(array=w166, index (row)=w167, index (col)=w169) -> (element=w172:T4)
      n78 = Bundle By Name(cluster=w172, "End Voltage"=w165) -> (w171:T4)
      n79 = Replace Array Subset(array=w163, new element=w171, index (row)=w167, index (col)=w169) -> (w170:T3)
      n80 = Bundle By Name(cluster=w174, "Red MOT 88 Inputs.Waveform Parameters"=w170) -> (w173:T1)
    }
    frame "ODT Params Final Voltage" {
      n81 = Unbundle By Name(w195) -> ("ODT Params.Waveform Parameters"=w187:T9[][])
      n82 = Increment(x=w190) -> (x+1=w189:dbl)
      n83 = case shown="True" w185 {
        tunnel: w187 -> [_ w203]
        tunnel: w186 -> [_ w202]
        tunnel: w188 -> [_ w198]
        tunnel: w189 -> [_ w199]
        tunnel: w187 -> [w196 w200]
        tunnel: [w196 w197] -> w184
        frame False {
        }
        frame True {
          n84 = Index Array(array=w203, index (row)=w198, index (col)=w199) -> (element=w204:T9)
          n85 = Bundle By Name(cluster=w204, "Initial Value"=w202) -> (w201:T9)
          n86 = Replace Array Subset(array=w200, new element=w201, index (row)=w198, index (col)=w199) -> (w197:T9[][])
        }
      }
      n87 = Index Array(array=w187, index (row)=w188, index (col)=w190) -> (element=w193:T9)
      n88 = Bundle By Name(cluster=w193, "Final Value"=w186) -> (w192:T9)
      n89 = Replace Array Subset(array=w184, new element=w192, index (row)=w188, index (col)=w190) -> (w191:T9[][])
      n90 = Bundle By Name(cluster=w195, "ODT Params.Waveform Parameters"=w191) -> (w194:T1)
    }
    frame "ODT Params Eta" {
      n91 = Unbundle By Name(w213) -> ("ODT Params.Waveform Parameters"=w208:T9[][])
      n92 = Index Array(array=w208, index (row)=w206, index (col)=w207) -> (element=w211:T9)
      n93 = Bundle By Name(cluster=w211, "Eta"=w210) -> (w209:T9)
      n94 = Replace Array Subset(array=w208, new element=w209, index (row)=w206, index (col)=w207) -> (w205:T9[][])
      n95 = Bundle By Name(cluster=w213, "ODT Params.Waveform Parameters"=w205) -> (w212:T1)
    }
    frame "PulseBlaster" {
      n96 = Unbundle By Name(w221) -> ("Instructions"=w215:T36)
      n97 = Index Array(array=w215, index=w216) -> (element=w218:T37)
      n98 = Bundle By Name(cluster=w218, "Time (s)"=w219) -> (w217:T37)
      n99 = Replace Array Subset(array=w215, new element=w217, index=w216) -> (w214:T36)
      n100 = Bundle By Name(cluster=w221, "Instructions"=w214) -> (w220:T1)
    }
    frame "Subroutine B Time" {
      n101 = Unbundle By Name(w229) -> ("Random Interleave Controls.Subroutine B"=w223:T36)
      n102 = Index Array(array=w223, index=w224) -> (element=w226:T37)
      n103 = Bundle By Name(cluster=w226, "Time (s)"=w227) -> (w225:T37)
      n104 = Replace Array Subset(array=w223, new element=w225, index=w224) -> (w222:T36)
      n105 = Bundle By Name(cluster=w229, "Random Interleave Controls.Subroutine B"=w222) -> (w228:T1)
    }
    frame "Subroutine A Time" {
      n106 = Unbundle By Name(w237) -> ("Random Interleave Controls.Subroutine A"=w231:T36)
      n107 = Index Array(array=w231, index=w232) -> (element=w234:T37)
      n108 = Bundle By Name(cluster=w234, "Time (s)"=w235) -> (w233:T37)
      n109 = Replace Array Subset(array=w231, new element=w233, index=w232) -> (w230:T36)
      n110 = Bundle By Name(cluster=w237, "Random Interleave Controls.Subroutine A"=w230) -> (w236:T1)
    }
    frame "Static Voltage" {
      n111 = Unbundle By Name(w243) -> ("6704 Static Voltage Settings.Values"=w241:dbl[])
      n112 = Replace Array Subset(array=w241, new element=w239, index=w240) -> (w238:dbl[])
      n113 = Bundle By Name(cluster=w243, "6704 Static Voltage Settings.Values"=w238) -> (w242:T1)
    }
    frame "Synth Phase" {
      n114 = Unbundle By Name(w246) -> ("Synth Controls.Channel Settings"=w247:T20[])
      n115 = Index Array(array=w247, index=w248) -> (element=w251:T20)
      n116 = Bundle By Name(cluster=w251, "Phase (deg)"=w250) -> (w249:T20)
      n117 = Replace Array Subset(array=w247, new element=w249, index=w248) -> (w245:T20[])
      n118 = Bundle By Name(cluster=w246, "Synth Controls.Channel Settings"=w245) -> (w244:T1)
    }
    frame "Synth Frequency" {
      n119 = Unbundle By Name(w254) -> ("Synth Controls.Channel Settings"=w255:T20[])
      n120 = Index Array(array=w255, index=w256) -> (element=w259:T20)
      n121 = Bundle By Name(cluster=w259, "Frequency (MHz)"=w258) -> (w257:T20)
      n122 = Replace Array Subset(array=w255, new element=w257, index=w256) -> (w253:T20[])
      n123 = Bundle By Name(cluster=w254, "Synth Controls.Channel Settings"=w253) -> (w252:T1)
    }
    frame "Synth Amplitude" {
      n124 = Unbundle By Name(w262) -> ("Synth Controls.Channel Settings"=w263:T20[])
      n125 = Index Array(array=w263, index=w264) -> (element=w267:T20)
      n126 = Bundle By Name(cluster=w267, "Voltage (Pk-Pk)"=w266) -> (w265:T20)
      n127 = Replace Array Subset(array=w263, new element=w265, index=w264) -> (w261:T20[])
      n128 = Bundle By Name(cluster=w262, "Synth Controls.Channel Settings"=w261) -> (w260:T1)
    }
  }
  "Spinal Column Out" <- w1
  n129 = case shown="\"Red Mot 88 Final Voltage\", Default" "What To Change" {
    tunnel: "Value" -> [w270 w273 w276 w279 w280]
    tunnel: [w268 w271 w274 w277 w280] -> _
    frame "PulseBlaster" {
      n130 = Multiply(x=w270, y=1000.0) -> (x*y=w268:dbl)
    }
    frame "ODT Params Phase Time" {
      n131 = Multiply(x=w273, y=1000.0) -> (x*y=w271:dbl)
    }
    frame "Red Mot 88 Phase Time" {
      n132 = Multiply(x=w276, y=1000.0) -> (x*y=w274:dbl)
    }
    frame "Red Mot 87 Phase Time" {
      n133 = Multiply(x=w279, y=1000.0) -> (x*y=w277:dbl)
    }
    frame "Red Mot 88 Final Voltage", Default {
    }
  }
